vi "CRYInsert Curve.vi"(8 "sOptionUpdate":string, 9 "sOption":string, 10 "Index":i32[](array[numeric]), 11 "Curve":T1 {"Z data" items=["dB", "Lin"]; "X data" items=["dB", "Lin"]; "Y data" items=["dB", "Lin"]; "Z dB ref" format="%.1f"; "Z axis" items=["Log", "Lin"]; "X dB ref" format="%.1f"; "X axis" items=["Log", "Lin"]; "Y axis" items=["Log", "Lin"]; "Y dB ref" format="%.1f"; "Curve"."z" format="%.2f"; "Curve"."y" format="%.2f"; "Curve"."x" format="%.2f"}) -> (2 "Inserted Index":i32[](array[numeric]), 3 "Inserted Name Out":string[](array[string]))   [LabVIEW 2013]
uses:
  CRYSystem/Typedef Control/CRYData Cluster Array.ctl
  CRYSystem/Typedef Control/CRYData Cluster.ctl
  Global/CRYCurve Library Global.vi
  CRYSystem/Task Sequence/CRYProject Run Control Global.vi
  Global/CRYCurves Array Global.vi
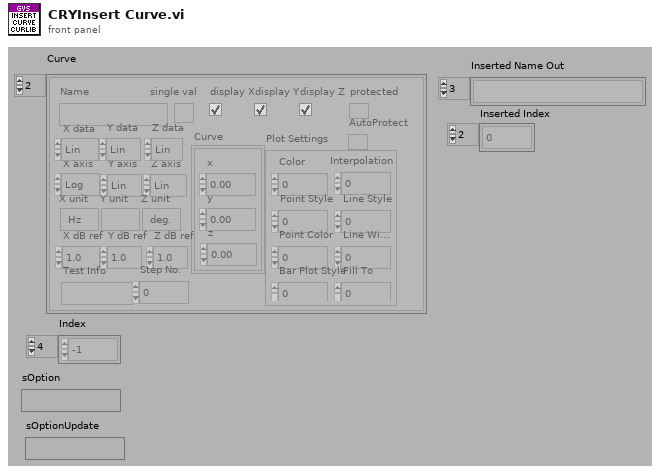
[diagram p1: front panel]
types:
  T1 = typedef "CRYData Cluster Array.ctl" = T2[]
  T2 = typedef "CRYData Cluster.ctl" = cluster{"Name":string, "Curve":cluster{"x":dbl, "y":dbl, "z":dbl}[], "X data":u16, "Y data":u16, "Z data":u16, "X axis":u16, "Y axis":u16, "Z axis":u16, "X unit":string, "Y unit":string, "Z unit":string, "X dB ref":dbl, "Y dB ref":dbl, "Z dB ref":dbl, "single val":bool, "protected":bool, "display X":bool, "display Y":bool, "display Z":bool, "Test Info":string, "Step No.":i32, "Plot Settings":cluster{"Color":u32, "Interpolation":u8, "Point Style":u8, "Line Style":u8, "Point Color":u32, "Line Width":u8, "Bar Plot Style":u8, "Fill To":i16}, "AutoProtect":bool}
  T3 = cluster{"CurveOld":string[], "ValueOld":string[], "ResultOld":string[], "WFMOld":string[], "CurveNew":string[], "ValueNew":string[], "ResultNew":string[], "WFMNew":string[]}
  T4 = cluster{"Color":u32, "Interpolation":u8, "Point Style":u8, "Line Style":u8, "Point Color":u32, "Line Width":u8, "Bar Plot Style":u8, "Fill To":i16}
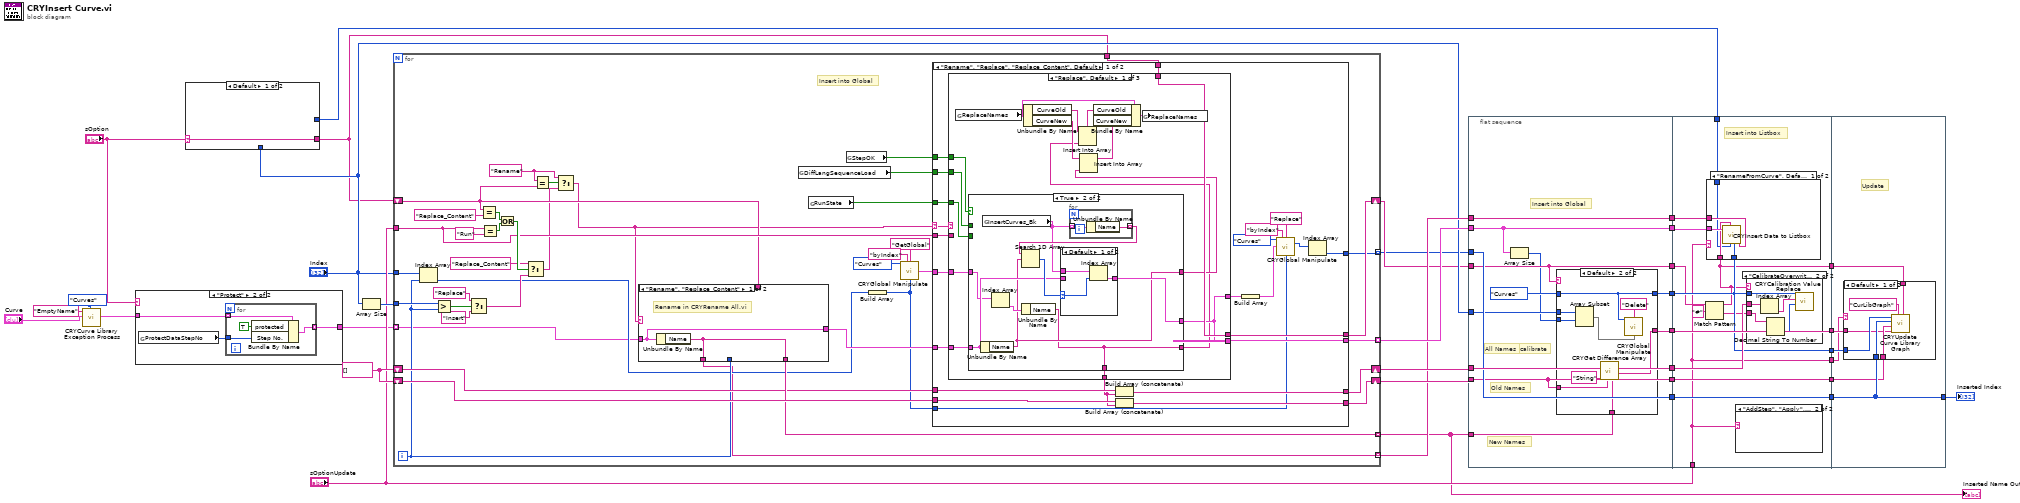
[diagram p0: block diagram]
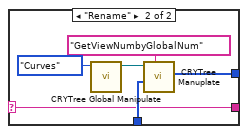
[diagram p3: hidden frame]
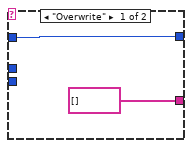
[diagram p4: hidden frame]
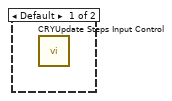
[diagram p5: hidden frame]
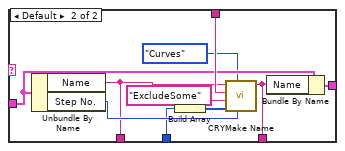
[diagram p9: hidden frame]
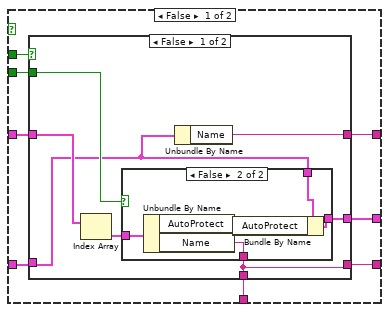
[diagram p10: hidden frame]
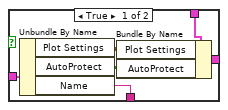
[diagram p11: hidden frame]
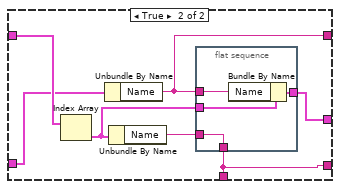
[diagram p12: hidden frame]
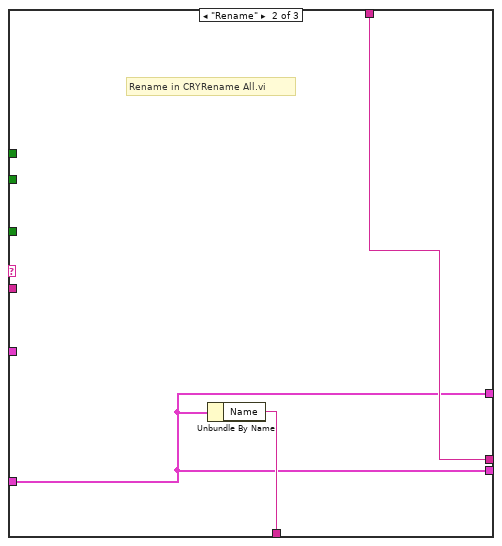
[diagram p14: hidden frame]
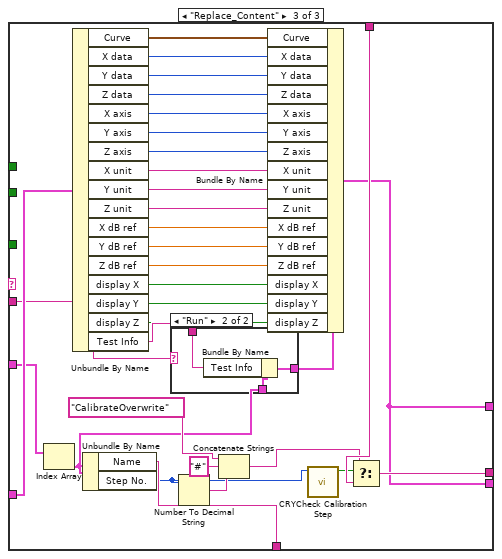
[diagram p15: hidden frame]
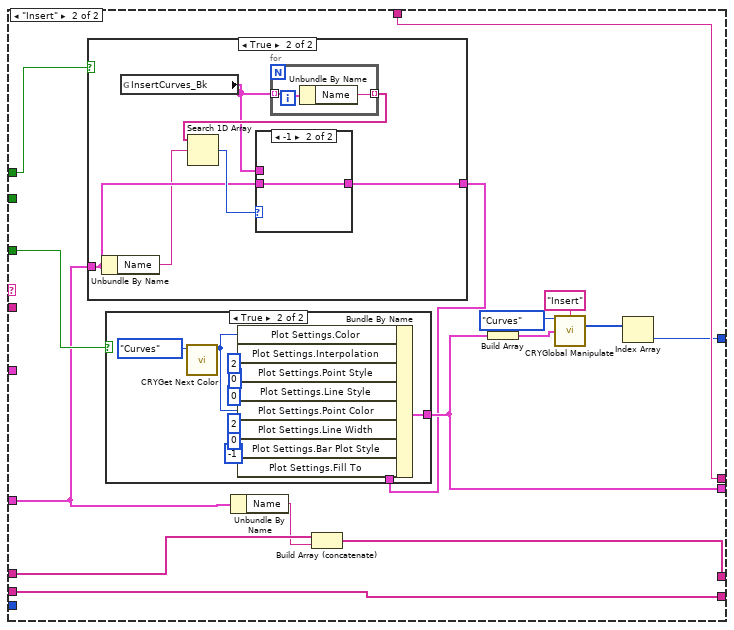
[diagram p17: hidden frame]
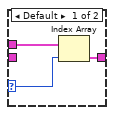
[diagram p19: hidden frame]
diagram:
  w22 = string[] []
  n1 = call "CRYCurve Library Exception Process.vi"("Type In"=enum16{"Curves", "Values", "Results", "WFM"}."Curves", "Curve/Value"="Curve", "sAction"="EmptyName") -> ("Curve/Value Out"=w1:T1)  [unwired: 6 in, 2 out]
  n2 = case shown="\"Protect\"" "sOption" {
    tunnel: w1 -> [w35 w38]
    tunnel: [w35 w37] -> w7
    frame Default {
    }
    frame "Protect" {
      n3 = global read "CRYCurve Library Global.vi" "ProtectDataStepNo"() -> (w36:i32)
      n4 = for {
        tunnel: w38 -> [w42] mode=indexing
        tunnel: [w41] -> w37 mode=indexing
        tunnel: w36 -> [w39]
        n5 = Bundle By Name(cluster=w42, "protected"=TRUE, "Step No."=w39) -> (w41:T2)
      }
    }
  }
  n6 = case shown="Default" "sOption" {
    selector: "sOption" -> [w43 w44]
    tunnel: "Index" -> [_ w45]
    tunnel: [_ w46] -> w10
    tunnel: [w43 w44] -> w11
    frame Default {
    }
    frame "Rename" {
      n7 = call "CRYTree Global Manipulate.vi"("Type In"=enum16{"Curves", "Values", "Results", "WFM"}."Curves") -> ("Tree/Curve Tree"=w47:refnum<vi>)  [unwired: 7 in, 3 out]
      n8 = call "CRYTree Manuplate.vi"("sAction"="GetViewNumbyGlobalNum", "nData"=w45, "Tree in"=w47) -> ("nData Out"=w46:i32[])  [unwired: 5 in, 3 out]
    }
  }
  n9 = Array Size(array="Index") -> (size(s)=w20:i32)
  n10 = for {
    tunnel: [w87] -> w5 mode=indexing
    tunnel: w7 -> [w51] mode=indexing
    tunnel: [w83] -> w15 mode=indexing
    tunnel: w20 -> [w77]
    shift-right: [w86] -> w23
    shift-left: w22 -> [w88]
    shift-right: [w84] -> w21
    shift-left: w22 -> [w85]
    tunnel: "Index" -> [w82]
    tunnel: w11 -> [w75]
    tunnel: "sOptionUpdate" -> [w67]
    tunnel: [w60] -> w14 mode=indexing
    shift-right: [w54] -> w9
    shift-left: w11 -> [w58]
    tunnel: [w52] -> w6 mode=indexing
    i -> [w73]
    w57 = "Rename" ("y")
    # "Insert into Global"
    n11 = Index Array(array=w82, index=w73) -> (element=w63:i32)
    n12 = Greater?(x=w77, y=w73) -> (0:w79:bool)
    n13 = Select(t="Replace" ("sOption"), s=w79, f="Insert" ("sOption")) -> (s? t:f=w78:string)
    n14 = Equal?(x=w58, y="Replace_Content") -> (x = y?=w71:bool)
    n15 = Equal?(x=w67, y="Run") -> (x = y?=w70:bool)
    n16 = Or(x=w71, y=w70) -> (x .or. y?=w69:bool)
    n17 = Select(t="Replace_Content" ("y"), s=w69, f=w78) -> (s? t:f=w56:string)
    n18 = Equal?(x=w57, y=w58) -> (x = y?=w59:bool)
    n19 = Select(t=w57, s=w59, f=w56) -> (s? t:f=w55:string)
    n20 = case shown="\"Rename\", \"Replace_Content\"" w55 {
      tunnel: [w91 w101] -> w89
      tunnel: [w90 w100] -> w87
      tunnel: w58 -> [_ w99]
      tunnel: w51 -> [w91 w98]
      tunnel: w73 -> [_ w93]
      tunnel: [w90 w92] -> w60
      frame "Rename", "Replace_Content" {
        # "Rename in CRYRename All.vi"
        n21 = Unbundle By Name(w91) -> ("Name"=w90:string)
      }
      frame Default {
        n22 = Unbundle By Name(w98) -> ("Name"=w92:string, "Step No."=w94:i32)
        n23 = Build Array(w93) -> (w96:i32[])
        n24 = call "CRYMake Name.vi"("Step No."=w94, "Type"=enum16{"Curves", "Values", "Results", "WFM"}."Curves", "nData"=w96, "sOption"="ExcludeSome", "sAction"=w99, "Name In"=w92) -> ("Name Out"=w100:string)  [unwired: 4 in, 1 out]
        n25 = Bundle By Name(cluster=w98, "Name"=w100) -> (w101:T2)
      }
    }
    n26 = global read "CRYCurve Library Global.vi" "DiffLangSequenceLoad"() -> (w53:bool)
    n27 = global read "CRYProject Run Control Global.vi" "RunState"() -> (w76:bool)
    n28 = global read "CRYCurve Library Global.vi" "StepOK"() -> (w50:bool)
    n29 = Build Array(w63) -> (w62:i32[])
    n30 = call "CRYGlobal Manipulate.vi"("Type"=enum16{"Curves", "Values", "Results", "WFM"}."Curves", "sOption"="byIndex", "sAction"="GetGlobal", "nData"=w62) -> ("Curves Out"=w65:T2[])  [unwired: 5 in, 6 out]
    n31 = case shown="\"Rename\", \"Replace\", \"Replace_Content\", Default" w55 {
      selector: w55 -> [w113 _]
      tunnel: w65 -> [w123 _]
      tunnel: w89 -> [w124 w233]
      tunnel: [w121 w246] -> w86
      tunnel: w88 -> [w122 w246]
      tunnel: w85 -> [w120 w245]
      tunnel: [w118 w243] -> w84
      tunnel: [w117 w238] -> w83
      tunnel: w76 -> [w116 w242]
      tunnel: w75 -> [w115 w241]
      tunnel: [w114 w241] -> w54
      tunnel: w67 -> [w112 _]
      tunnel: w62 -> [w107 _]
      tunnel: w53 -> [w105 _]
      tunnel: [w103 w235] -> w52
      tunnel: w50 -> [w102 w234]
      frame "Rename", "Replace", "Replace_Content", Default {
        n32 = case shown="\"Replace\", Default" w113 {
          tunnel: w124 -> [w138 w193 w226]
          tunnel: w123 -> [w140 _ w200]
          tunnel: [w139 w194 w227] -> w119
          tunnel: [w135 w193 w201] -> w117
          tunnel: w116 -> [w137 _ _]
          tunnel: w115 -> [w136 w195 w215]
          tunnel: [w136 w195 w214] -> w114
          tunnel: w112 -> [_ _ w204]
          tunnel: [w135 w193 w201] -> w109
          tunnel: w105 -> [w134 _ _]
          tunnel: w102 -> [w125 _ _]
          frame "Replace", Default {
            n33 = global read "CRYCurve Library Global.vi" "ReplaceNames"() -> (w133:T3)
            n34 = case shown="True" w125 {
              tunnel: w140 -> [w148 w181]
              tunnel: [w147 w178] -> w139
              tunnel: w138 -> [w146 w183]
              tunnel: w137 -> [w145 _]
              tunnel: [w144 w182] -> w135
              tunnel: w134 -> [w143 _]
              tunnel: [w142 w179] -> w129
              tunnel: [w141 w178] -> w128
              frame False {
                n35 = case shown="False" w143 {
                  tunnel: w148 -> [w154 w173]
                  tunnel: [w149 w168] -> w147
                  tunnel: w146 -> [w151 w171]
                  tunnel: w145 -> [w153 _]
                  tunnel: [w152 w172] -> w144
                  tunnel: [w150 w167] -> w142
                  tunnel: [w149 w168] -> w141
                  frame False {
                    n36 = Index Array(array=w154) -> (element=w155:T2)  [unwired: 1 in]
                    n37 = case shown="False" w153 {
                      tunnel: w155 -> [w161 w166]
                      tunnel: [w160 w165] -> w149
                      tunnel: w151 -> [w158 w163]
                      tunnel: [w157 w162] -> w152
                      frame True {
                        n38 = Unbundle By Name(w161) -> ("Plot Settings"=w156:T4, "AutoProtect"=w159:bool, "Name"=w160:string)
                        n39 = Bundle By Name(cluster=w158, "Plot Settings"=w156, "AutoProtect"=w159) -> (w157:T2)
                      }
                      frame False {
                        n40 = Unbundle By Name(w166) -> ("AutoProtect"=w164:bool, "Name"=w165:string)
                        n41 = Bundle By Name(cluster=w163, "AutoProtect"=w164) -> (w162:T2)
                      }
                    }
                    n42 = Unbundle By Name(w151) -> ("Name"=w150:string)
                  }
                  frame True {
                    n43 = Index Array(array=w173) -> (element=w170:T2)  [unwired: 1 in]
                    n44 = Unbundle By Name(w171) -> ("Name"=w167:string)
                    n45 = Unbundle By Name(w170) -> ("Name"=w169:string)
                    n46 = flat-sequence {
                      tunnel: [w177] -> w172
                      tunnel: w167 -> [w176]
                      tunnel: w170 -> [w175]
                      tunnel: [w174] -> w168
                      tunnel: w169 -> [w174]
                      frame #0 {
                        n47 = Bundle By Name(cluster=w175, "Name"=w176) -> (w177:T2)
                      }
                    }
                  }
                }
              }
              frame True {
                n48 = Unbundle By Name(w183) -> ("Name"=w179:string)
                n49 = global read "CRYCurves Array Global.vi" "InsertCurves_Bk"() -> (w184:T1)
                n50 = Index Array(array=w181) -> (element=w180:T2)  [unwired: 1 in]
                n51 = Unbundle By Name(w180) -> ("Name"=w178:string)
                n52 = for {
                  tunnel: w184 -> [w192] mode=indexing
                  tunnel: [w191] -> w186 mode=indexing
                  n53 = Unbundle By Name(w192) -> ("Name"=w191:string)
                }
                n54 = Search 1D Array(1D array=w186, element=w179) -> (index of element=w185:i32)  [unwired: 1 in]
                n55 = case shown="Default" w185 {
                  selector: w185 -> [w188 _]
                  tunnel: w184 -> [w189 _]
                  tunnel: [w187 w190] -> w182
                  tunnel: w183 -> [_ w190]
                  frame Default {
                    n56 = Index Array(array=w189, index=w188) -> (element=w187:T2)
                  }
                  frame -1 {
                  }
                }
              }
            }
            n57 = Unbundle By Name(w133) -> ("CurveOld"=w131:string[], "CurveNew"=w130:string[])
            n58 = Insert Into Array(array=w131, new element=w128) -> (w127:string[])  [unwired: 1 in]
            n59 = Insert Into Array(array=w130, new element=w129) -> (w126:string[])  [unwired: 1 in]
            n60 = Bundle By Name(cluster=w133, "CurveOld"=w127, "CurveNew"=w126) -> (w132:T3)
            n61 = global write "CRYCurve Library Global.vi" "ReplaceNames"(w132) -> ()
          }
          frame "Rename" {
            # "Rename in CRYRename All.vi"
            n62 = Unbundle By Name(w193) -> ("Name"=w194:string)
          }
          frame "Replace_Content" {
            n63 = Index Array(array=w200) -> (element=w203:T2)  [unwired: 1 in]
            n64 = Unbundle By Name(w226) -> ("Curve"=w225:cluster{"x":dbl, "y":dbl, "z":dbl}[], "X data"=w224:u16, "Y data"=w223:u16, "Z data"=w222:u16, "X axis"=w221:u16, "Y axis"=w220:u16, "Z axis"=w219:u16, "X unit"=w218:string, "Y unit"=w217:string, "Z unit"=w216:string, "X dB ref"=w207:dbl, "Y dB ref"=w206:dbl, "Z dB ref"=w205:dbl, "display X"=w198:bool, "display Y"=w197:bool, "display Z"=w196:bool, "Test Info"=w199:string)
            n65 = Unbundle By Name(w203) -> ("Name"=w227:string, "Step No."=w210:i32)
            n66 = case shown="\"Run\"" w204 {
              tunnel: w203 -> [w228 w231]
              tunnel: [w228 w230] -> w202
              tunnel: w199 -> [_ w229]
              frame Default {
              }
              frame "Run" {
                n67 = Bundle By Name(cluster=w231, "Test Info"=w229) -> (w230:T2)
              }
            }
            n68 = Number To Decimal String(number=w210) -> (decimal integer string=w212:string)  [unwired: 1 in]
            n69 = Concatenate Strings("CalibrateOverwrite" ("f"), "#" ("string"), w212) -> (w208:string)
            n70 = Bundle By Name(cluster=w202, "Curve"=w225, "X data"=w224, "Y data"=w223, "Z data"=w222, "X axis"=w221, "Y axis"=w220, "Z axis"=w219, "X unit"=w218, "Y unit"=w217, "Z unit"=w216, "X dB ref"=w207, "Y dB ref"=w206, "Z dB ref"=w205, "display X"=w198, "display Y"=w197, "display Z"=w196) -> (w201:T2)
            n71 = call "CRYCheck Calibration Step.vi"("Step No"=w210) -> ("Is Calibration?"=w213:bool)  [unwired: 9 in, 1 out]
            n72 = Select(t=w208, s=w213, f=w215) -> (s? t:f=w214:string)
          }
        }
        n73 = Build Array (concatenate)(w120, w119) -> (w118:string[])
        n74 = Build Array (concatenate)(w122, w119) -> (w121:string[])
        n75 = Build Array(w109) -> (w108:T2[])
        n76 = call "CRYGlobal Manipulate.vi"("Type"=enum16{"Curves", "Values", "Results", "WFM"}."Curves", "sOption"="byIndex", "sAction"="Replace", "Curves"=w108, "nData"=w107) -> ("nData out"=w104:i32[])  [unwired: 4 in, 6 out]
        n77 = Index Array(array=w104) -> (element=w103:i32)  [unwired: 1 in]
      }
      frame "Insert" {
        n78 = case shown="True" w234 {
          tunnel: w233 -> [w247 w250]
          tunnel: [w247 w249] -> w232
          frame False {
          }
          frame True {
            n79 = Unbundle By Name(w250) -> ("Name"=w248:string)
            n80 = global read "CRYCurves Array Global.vi" "InsertCurves_Bk"() -> (w251:T1)
            n81 = for {
              tunnel: w251 -> [w259] mode=indexing
              tunnel: [w258] -> w253 mode=indexing
              n82 = Unbundle By Name(w259) -> ("Name"=w258:string)
            }
            n83 = Search 1D Array(1D array=w253, element=w248) -> (index of element=w252:i32)  [unwired: 1 in]
            n84 = case shown="-1" w252 {
              selector: w252 -> [w255 _]
              tunnel: w251 -> [w256 _]
              tunnel: [w254 w257] -> w249
              tunnel: w250 -> [_ w257]
              frame Default {
                n85 = Index Array(array=w256, index=w255) -> (element=w254:T2)
              }
              frame -1 {
              }
            }
          }
        }
        n86 = case shown="True" w242 {
          tunnel: w232 -> [w260 w263]
          tunnel: [w260 w262] -> w238
          frame False {
          }
          frame True {
            n87 = call "CRYGet Next Color.vi"("Type"=enum16{"Curves", "Values", "Results", "WFM"}."Curves") -> ("Color"=w267:u32)  [unwired: 10 out]
            n88 = Bundle By Name(cluster=w263, "Plot Settings.Color"=w267, "Plot Settings.Interpolation"=u8 2, "Plot Settings.Point Style"=u8 0, "Plot Settings.Line Style"=u8 0, "Plot Settings.Point Color"=w267, "Plot Settings.Line Width"=u8 2, "Plot Settings.Bar Plot Style"=u8 0, "Plot Settings.Fill To"=i16 -1) -> (w262:T2)
          }
        }
        n89 = Unbundle By Name(w233) -> ("Name"=w244:string)
        n90 = Build Array (concatenate)(w245, w244) -> (w243:string[])
        n91 = Build Array(w238) -> (w237:T2[])
        n92 = call "CRYGlobal Manipulate.vi"("Type"=enum16{"Curves", "Values", "Results", "WFM"}."Curves", "sAction"="Insert", "Curves"=w237) -> ("nData out"=w236:i32[])  [unwired: 6 in, 6 out]
        n93 = Index Array(array=w236) -> (element=w235:i32)  [unwired: 1 in]
      }
    }
  }
  "Inserted Name Out" <- w5
  n94 = flat-sequence {
    tunnel: [w276] -> w32
    tunnel: w15 -> [w276]
    tunnel: "Index" -> [w274]
    tunnel: w23 -> [w272]
    tunnel: [w282] -> w33
    tunnel: [w272] -> w34
    tunnel: [w281] -> w31
    tunnel: [w277] -> w30
    tunnel: [w279] -> w29
    tunnel: w21 -> [w279]
    tunnel: w9 -> [w275]
    tunnel: [w275] -> w28
    tunnel: w14 -> [w278]
    tunnel: [w278] -> w13
    tunnel: w6 -> [w277]
    tunnel: w5 -> [w271]
    tunnel: [w306] -> w27
    tunnel: [w305] -> w26
    tunnel: w34 -> [w305]
    tunnel: w33 -> [w306]
    tunnel: w32 -> [w304]
    tunnel: w31 -> [w301]
    tunnel: [w301] -> w25
    tunnel: w30 -> [w303]
    tunnel: [w303] -> w24
    tunnel: w29 -> [w302]
    tunnel: w28 -> [w297]
    tunnel: [w294] -> w18
    tunnel: [w295] -> w17
    tunnel: "sOptionUpdate" -> [w294]
    tunnel: w13 -> [w298]
    tunnel: w10 -> [w296]
    tunnel: w27 -> [w319]
    tunnel: w26 -> [w320]
    tunnel: w25 -> [w322]
    tunnel: w24 -> [w321]
    tunnel: [w321] -> w19
    tunnel: w18 -> [w318]
    tunnel: w17 -> [w317]
    frame #0 {
      # "New Names"
      # "Insert into Global"
      # "All Names"
      # "calibrate"
      # "Old Names"
      n95 = Array Size(array=w276) -> (size(s)=w273:i32)
      n96 = case shown="Default" w275 {
        tunnel: [string[] [] ("Deleted Names") w286] -> w282
        tunnel: [w284 w292] -> w281
        tunnel: enum16{"Curves", "Values", "Results", "WFM"}."Curves" ("Type") -> [w284 w292]
        tunnel: w274 -> [_ w291]
        tunnel: w273 -> [_ w290]
        tunnel: w272 -> [_ w288]
        tunnel: w271 -> [_ w287]
        frame "Overwrite" {
        }
        frame Default {
          n97 = Array Subset(array=w291, index=w290) -> (w289:i32[])  [unwired: 1 in]
          n98 = call "CRYGet Difference Array.vi"("String2"=w287, "String1"=w288, "sOption"="String") -> ("StringDiff Out"=w286:string[])  [unwired: 7 in, 1 out]
          n99 = call "CRYGlobal Manipulate.vi"("Type"=w292, "sAction"="Delete", "nData"=w289) -> ()  [unwired: 6 in, 7 out]
        }
      }
    }
    frame #1 {
      # "Insert into Listbox"
      n100 = Match Pattern(string=w297, regular expression="#" ("string")) -> (before substring=w295:string, after substring=w299:string)  [unwired: 1 in, 2 out]
      n101 = case shown="\"RenameFromCurve\", Default" w294 {
        tunnel: w304 -> [w311 _]
        tunnel: w301 -> [w310 _]
        tunnel: w298 -> [w309 _]
        tunnel: w295 -> [w308 _]
        tunnel: w296 -> [w307 _]
        frame "RenameFromCurve", Default {
          n102 = call "CRYInsert Data to Listbox.vi"("OrgNames"=w309, "Type"=w310, "nData"=w307, "sOption"=w308, "Curves"=w311) -> ()  [unwired: 6 in, 1 out]
        }
        frame "Run" {
        }
      }
      n103 = case shown="\"AddStep\", \"Apply\", \"Run\"" w294 {
        frame Default {
          n104 = call "CRYUpdate Steps Input Control.vi"() -> ()  [unwired: 12 in]
        }
        frame "AddStep", "Apply", "Run" {
        }
      }
      n105 = case shown="\"CalibrateOverwrite\"" w295 {
        tunnel: w302 -> [_ w315]
        tunnel: w301 -> [_ w314]
        tunnel: w299 -> [_ w313]
        frame Default {
        }
        frame "CalibrateOverwrite" {
          n106 = Index Array(array=w315) -> (element=w316:string)  [unwired: 1 in]
          n107 = Decimal String To Number(string=w313) -> (number=w312:i32)  [unwired: 2 in, 1 out]
          n108 = call "CRYCalibration Value Replace.vi"("Step No."=w312, "Corr/EQ/Sens Name"=w316, "Type"=w314) -> ()  [unwired: 9 in]
        }
      }
    }
    frame #2 {
      # "Update"
      n109 = case shown="Default" w318 {
        tunnel: w322 -> [w327 _]
        tunnel: w321 -> [w326 _]
        tunnel: w320 -> [w325 _]
        tunnel: w319 -> [w323 _]
        tunnel: w317 -> [w324 _]
        frame Default {
          n110 = call "CRYUpdate Curve Library Graph.vi"("sOption 2"=w324, "sOption 1"="CurLibGraph" ("sOption"), "Deleted Names"=w323, "Replaced Old Names"=w325, "Index"=w326, "Type"=w327) -> ()  [unwired: 6 in]
        }
        frame "RenameFromCurve", "Run" {
        }
      }
    }
  }
  "Inserted Index" <- w19
